vi "ZurichAE.vi"(7 "zi Address":string="DEV1925", 8 "Y gain":dbl, 9 "X gain":dbl, 10 "V oscillation":dbl, 11 "Action":T1=enum."Close") -> (0 "Zurich Errors":errorcluster)   [LabVIEW 2022 SP3]
uses:
  Control_ZurichAE.ctl
  <instrlib>/Zurich Instruments LabOne/Public/Configure/ziSetValueDouble.vi
  <instrlib>/Zurich Instruments LabOne/Zurich Instruments LabOne.lvlib
panel:
  in  "Aux Y- address":string="auxouts/2/scale"
  in  "Aux Y+ address":string="auxouts/0/scale"
  in  "Aux X- address":string="auxouts/3/scale"
  in  "Aux X+ address":string="auxouts/1/scale"
  in  "Slow wiggler osc address":string="demods/4/oscselect/"
  in  "Slow wiggler amp address":string="sigouts/0/amplitudes/4"
  in  "Slow wiggler enable address":string="sigouts/0/enables/4"
  in  "Fast wiggler amp address":string="sigouts/0/amplitudes/7"
  # "Auxouts are usually configured as:\n0: Y+ (+M)\n1: X+ (+2M)\n2: Y- (-M)\n3: X- (-2M)"
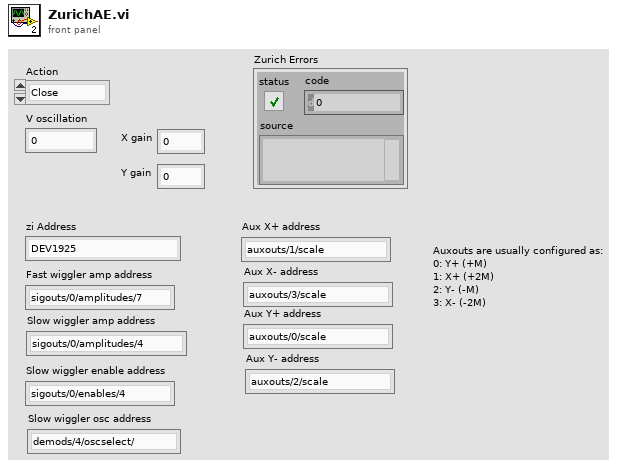
[diagram p1: front panel]
types:
  T1 = typedef "Control_ZurichAE.ctl" = enum16{"Initialize", "Set V oscillation", "Set XY gains", "Close", "Done"}
  T2 = typedef "Zurich Instruments LabOne.lvlib/ziTypeHandle.ctl" = cluster{"handleValid":bool, "Conn":u64, "Path Prefix":string, "Handle":u64, "Connected":bool, "Clockbase(s)":dbl}
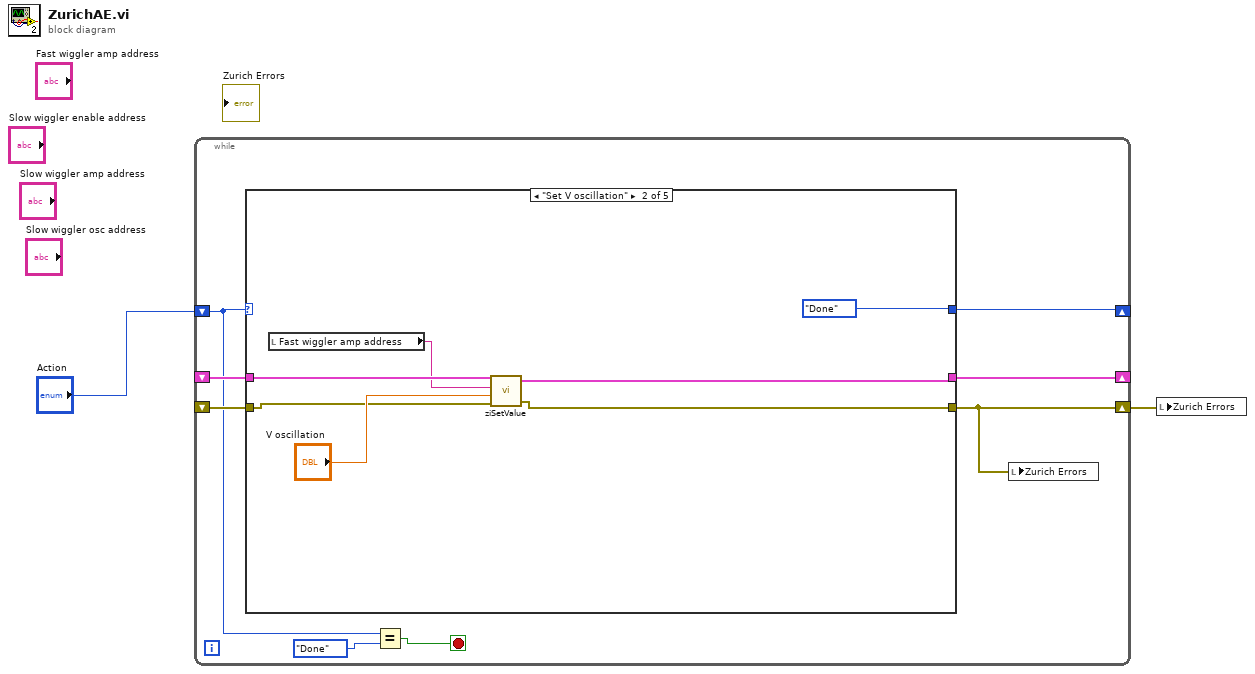
[diagram p0: block diagram]
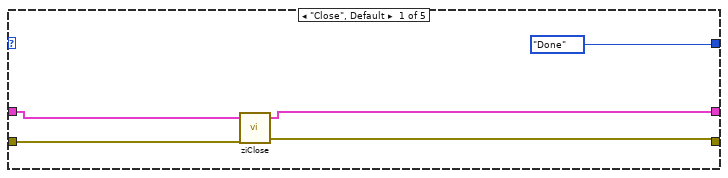
[diagram p2: hidden frame]
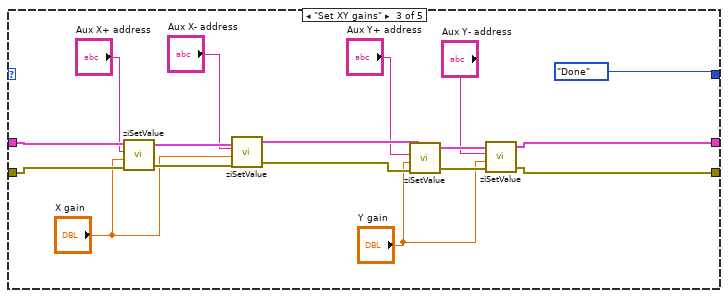
[diagram p3: hidden frame]
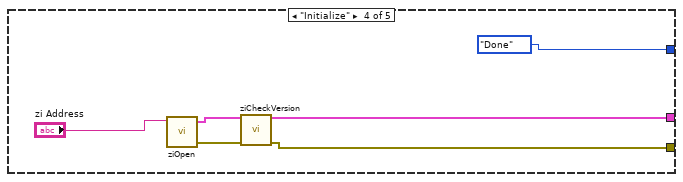
[diagram p4: hidden frame]
diagram:
  n1 = while {
    shift-right: [w10] -> _
    shift-left: _ -> [w9]
    shift-right: [w7] -> w1
    shift-left: _ -> [w8]
    shift-right: [w3] -> _
    shift-left: "Action" -> [w4]
    stop <- w6 stop-if-true
    n2 = case shown="\"Set V oscillation\"" w4 {
      selector: w4 -> [_ _ _ _ w46]
      tunnel: [w13 w18 w34 w42 w48] -> w10
      tunnel: [w12 w17 w30 w41 w47] -> w7
      tunnel: w9 -> [w15 w21 w39 _ w48]
      tunnel: w8 -> [w14 w19 w38 _ w47]
      tunnel: [Control_ZurichAE."Done" ("Enum") Control_ZurichAE."Done" ("Enum") Control_ZurichAE."Done" ("Enum") Control_ZurichAE."Done" ("Enum") w46] -> w3
      frame "Close", Default {
        n3 = call <instrlib>:"ziClose.vi"("Error In"=w14, "Handle In"=w15) -> ("Error Out"=w12:errorcluster, "Handle Out"=w13:T2)  [unwired: 2 out]
      }
      frame "Set V oscillation" {
        n4 = local read "Fast wiggler amp address"() -> (w20:string)
        n5 = call-poly <instrlib>:"ziSetValue.vi"("Error In"=w19, "Value"="V oscillation", "Path"=w20, "Handle In"=w21) -> ("Error Out"=w17:errorcluster, "Handle Out"=w18:T2)  [unwired: 1 in]
      }
      frame "Set XY gains" {
        n6 = call-poly <instrlib>:"ziSetValue.vi"("Error In"=w38, "Value"="X gain", "Path"="Aux X+ address", "Handle In"=w39) -> ("Error Out"=w33:errorcluster, "Handle Out"=w37:T2)  [unwired: 1 in]
        n7 = call-poly <instrlib>:"ziSetValue.vi"("Error In"=w33, "Value"="X gain", "Path"="Aux X- address", "Handle In"=w37) -> ("Error Out"=w32:errorcluster, "Handle Out"=w36:T2)  [unwired: 1 in]
        n8 = call-poly <instrlib>:"ziSetValue.vi"("Error In"=w32, "Value"="Y gain", "Path"="Aux Y+ address", "Handle In"=w36) -> ("Error Out"=w31:errorcluster, "Handle Out"=w35:T2)  [unwired: 1 in]
        n9 = call-poly <instrlib>:"ziSetValue.vi"("Error In"=w31, "Value"="Y gain", "Path"="Aux Y- address", "Handle In"=w35) -> ("Error Out"=w30:errorcluster, "Handle Out"=w34:T2)  [unwired: 1 in]
      }
      frame "Initialize" {
        n10 = call <instrlib>:"ziOpen.vi"("Address"="zi Address") -> ("Error Out"=w45:errorcluster, "HandleOut"=w43:T2)  [unwired: 1 in, 3 out]
        n11 = call <instrlib>:"ziCheckVersion.vi"("Handle In"=w43, "Error In"=w45) -> ("Handle Out"=w42:T2, "Error Out"=w41:errorcluster)  [unwired: 11 in, 1 out]
      }
      frame "Done" {
      }
    }
    n12 = Equal?(x=w4, y=Control_ZurichAE."Done" ("Enum")) -> (x = y?=w6:bool)
    n13 = local write "Zurich Errors"(w7) -> ()
  }
  n14 = local write "Zurich Errors"(w1) -> ()
